vi "读取图像文件.vi"() -> ()   [LabVIEW 2010]
panel:
  out "图片2":picture
  out "图片":picture
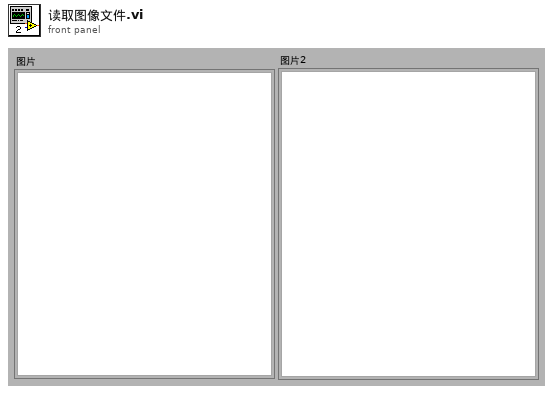
[diagram p1: front panel]
types:
  T1 = typedef "imagedata.ctl" = cluster{"image type":i32, "image depth":i32, "image":u8[], "mask":u8[], "colors":u32[], "Rectangle":cluster{"left":i16, "top":i16, "right":i16, "bottom":i16}}
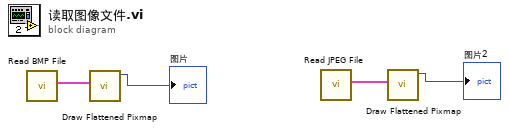
[diagram p0: block diagram]
diagram:
  n1 = call <vilib>:"Read BMP File.vi"() -> ("image data"=w4:T1)  [unwired: 9 in, 2 out]
  n2 = call <vilib>:"Draw Flattened Pixmap.vi"("image data"=w4) -> ("new picture"=→"图片":picture)  [unwired: 8 in]
  n3 = call <vilib>:"Read JPEG File.vi"() -> ("image data"=w2:T1)  [unwired: 9 in, 2 out]
  n4 = call <vilib>:"Draw Flattened Pixmap.vi"("image data"=w2) -> ("new picture"=→"图片2":picture)  [unwired: 8 in]
